vi "PiezoController main.vi"(10 "Top":refnum<queue>, 11 "Rotator":refnum<queue>) -> (3 "Ended":bool)   [LabVIEW 2022 SP3, in "SampleRotator.lvlib"]
doc: "This is a main VI of module for Sample rotator. It recives and executes commands, which comes from master controller. \nCommands and responses:\n\n/* */\nInitialize(path to driver DLL); -> Initialized(Contoller info<devN, devT, ID, Serial, Addr, connected?>);\n\n/* */\nUpdate(); -> Update(axis status<axis info, position, frequency, voltage>);\n\n/* */\nSetParameters(parameters<freq[Hz]; ampl[V]; offset[V]; tolerance[um]>); -> ParametersSet(parameters<freq; amp; offset; tolerance>);\n\n/* */\nSetPositon(positionToSet<relative?, double>) -> PositionSet(position to set<relative?, doubele);\n\n/* */\nEnd(), -> Disconnected();"
uses:
  SampleRotator.lvlib
  ctl/Rotator all.ctl
  ctl/Axis status.ctl
  Messenger service/Data types/Module name.ctl
  ctl/Motion Properties.ctl
  ctl/Positoin to set.ctl
  ctl/Rotator commands.ctl
panel:
  out "Piezo\nstatus":T1 {"Axes"."Index" items=["1", "2", "3"]; "Axes"."ActuatorType" items=["Linear", "Rotator", "Goniometer"]; "Features" format="%08b"; "FW-Version" format="%x"; "Controller info"."DeviceType" items=["ANC350res", "ANC350num", "ANC350fps", "No device / invalid"]; "Controller info"."ID" format="%x"}
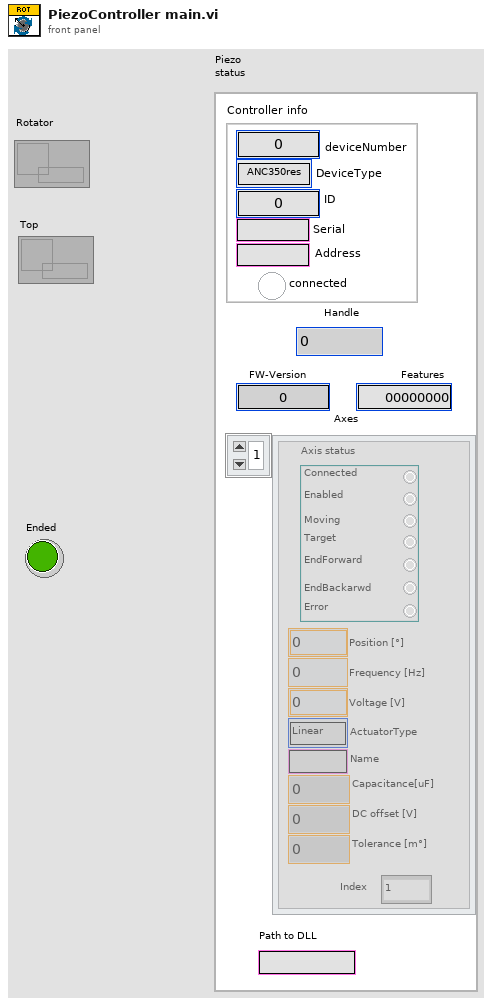
[diagram p1: front panel]
types:
  T1 = typedef "SampleRotator.lvlib/Rotator all.ctl" = cluster{"Controller info":cluster{"deviceNumber":i32, "DeviceType":i32, "ID":u32, "Serial":string, "Address":string, "connected":bool}, "Handle":u64, "FW-Version":i32, "Features":u32, "Axes":T2[], "Path to DLL":path}
  T2 = typedef "SampleRotator.lvlib/Axis status.ctl" = cluster{"Axis status":cluster{"Connected":bool, "Enabled":bool, "Moving":bool, "Target":bool, "EndForward":bool, "EndBackarwd":bool, "Error":bool}, "Position [°]":dbl, "Frequency [Hz]":dbl, "Voltage [V]":dbl, "Capacitance[uF]":dbl, "Name":string, "ActuatorType":u16, "DC offset [V]":dbl, "Tolerance [m°]":dbl, "Index":u8}
  T3 = typedef "SampleRotator.lvlib/Rotator commands.ctl" = enum16{"Ignore", "Initialize", "Initialize axes", "Update", "Set parameters", "Stop movement", "Set position", "Disconnect", "End"}
  T4 = typedef "Module name.ctl" = enum16{"Emty", "Magnet", "VTI", "Excitation", "Servo", "Acquisition", "Rotator", "Digitizer", "SMU2450", "Carousel", "Multimeter", "Tmp monitor", "Power monitor"}
  T5 = typedef "Motion Properties.ctl" = cluster{"Frequency [Hz]":dbl, "MaxErr [µm|m°]":dbl, "DC voltage [V]":dbl, "Amplitude [V]":dbl, "Position [mm|°]":dbl, "EoF":bool, "EoB":bool, "Error":bool, "Target [mm|°]":dbl}
  T6 = typedef "Positoin to set.ctl" = cluster{"Relative?":bool, "Position [°]":dbl, "Safe to move?":bool}
  T7 = cluster{"deviceNumber":i32, "DeviceType":i32, "ID":u32, "Serial":string, "Address":string, "connected":bool}
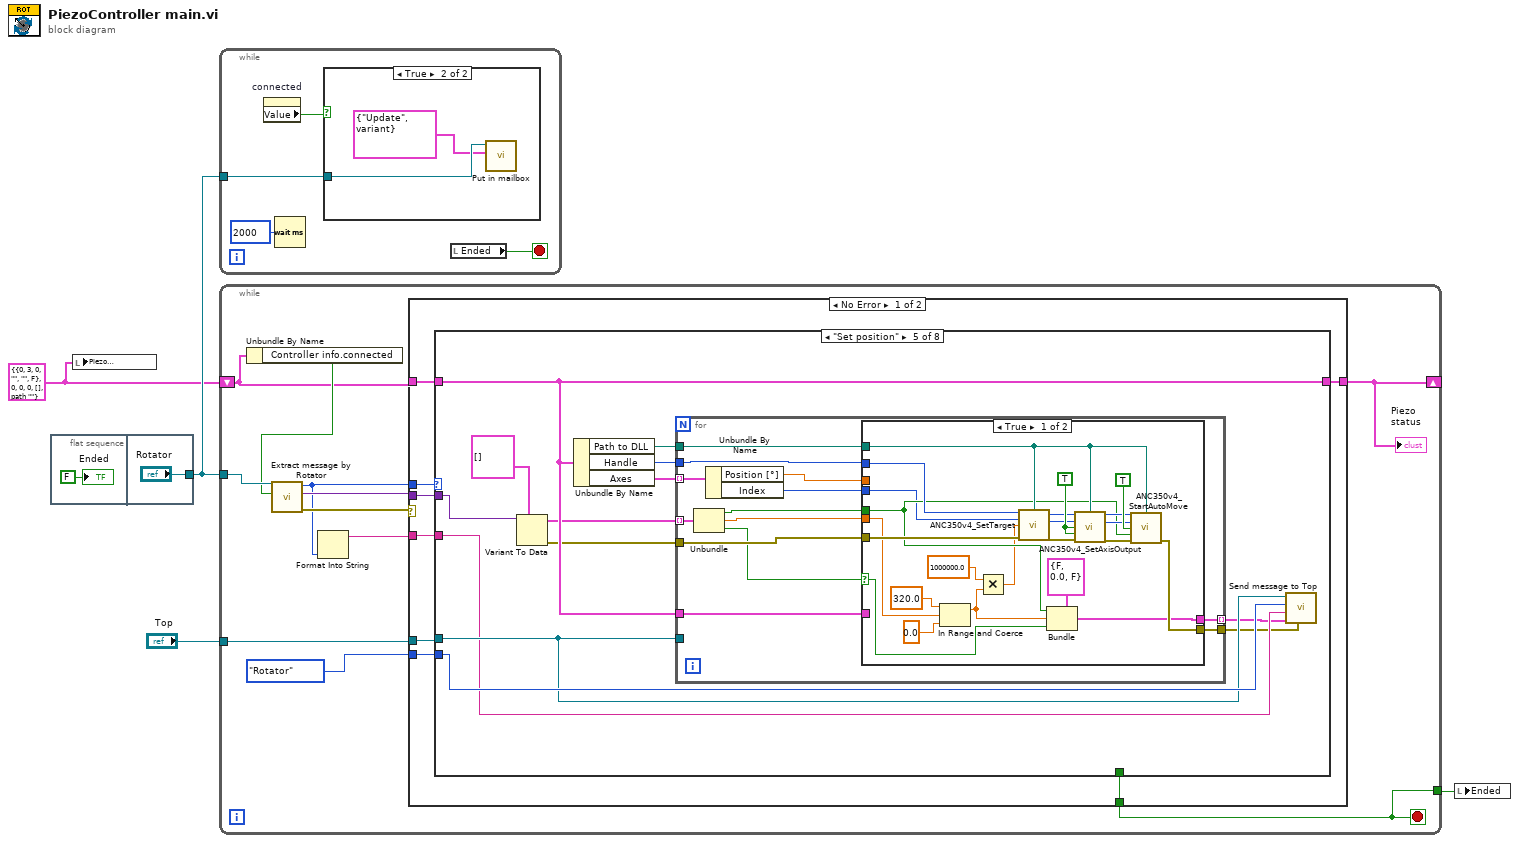
[diagram p0: block diagram]
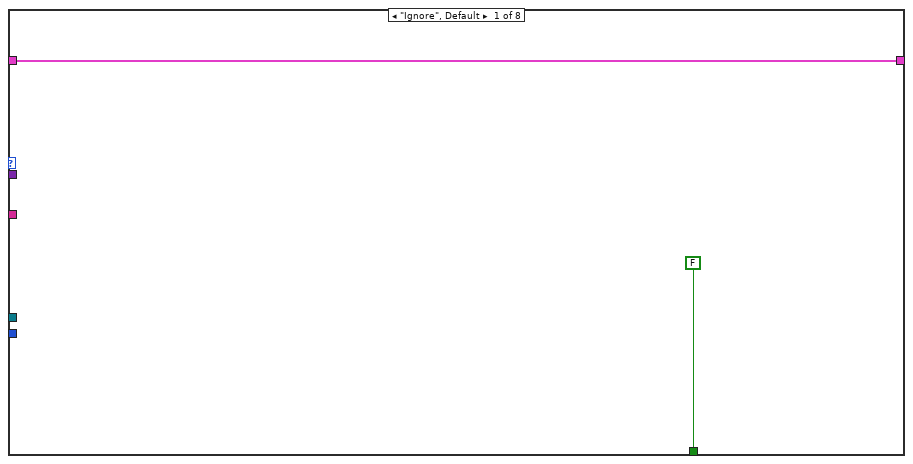
[diagram p3: hidden frame]
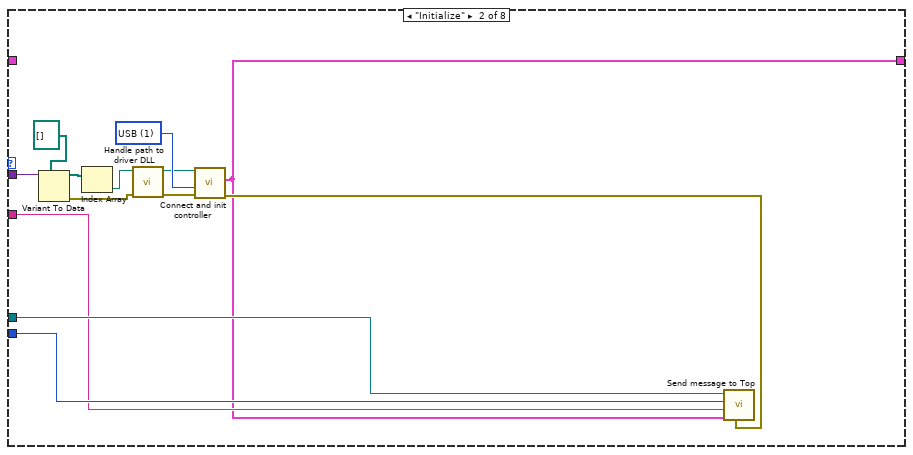
[diagram p4: hidden frame]
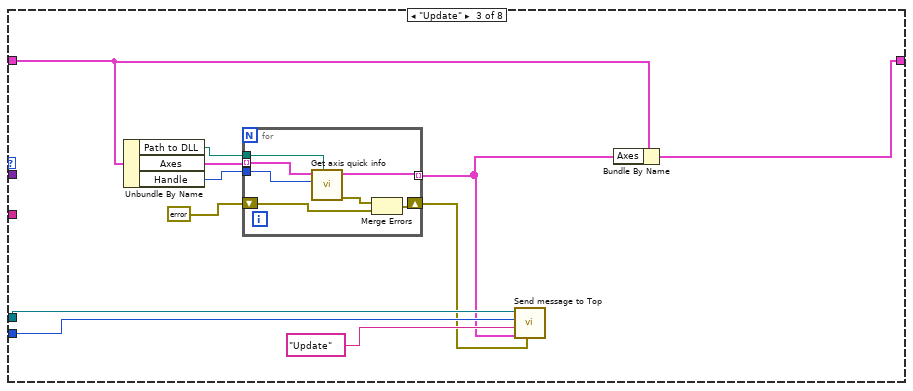
[diagram p5: hidden frame]
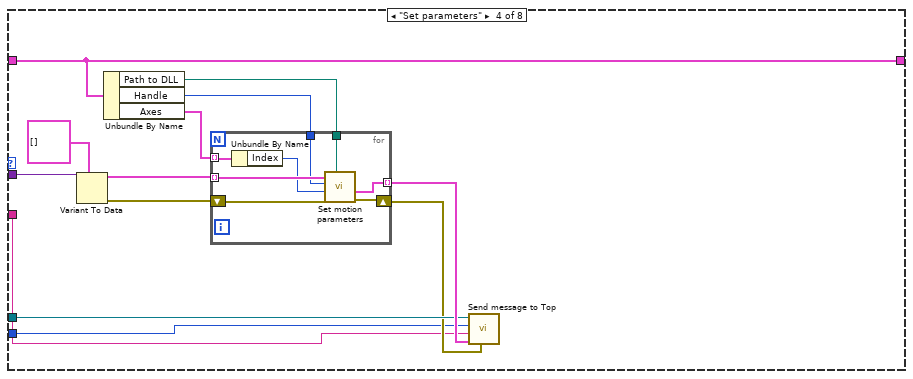
[diagram p6: hidden frame]
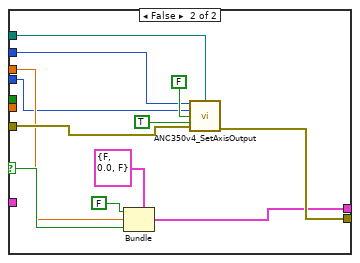
[diagram p7: hidden frame]
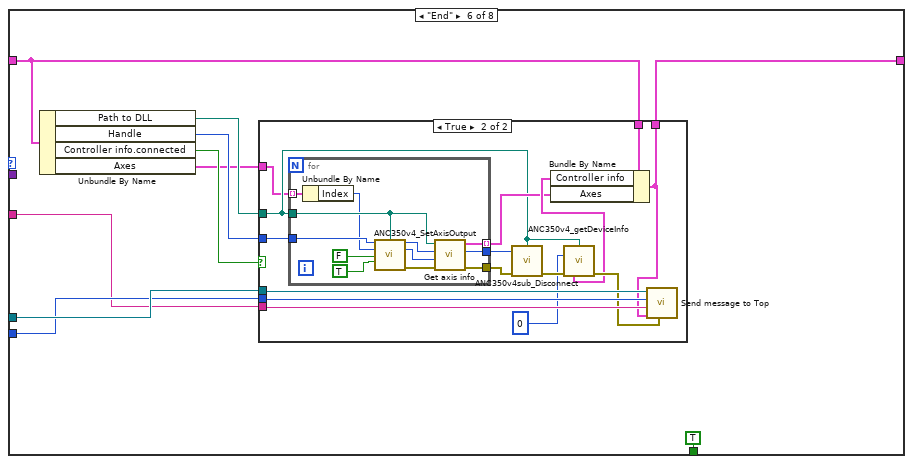
[diagram p8: hidden frame]
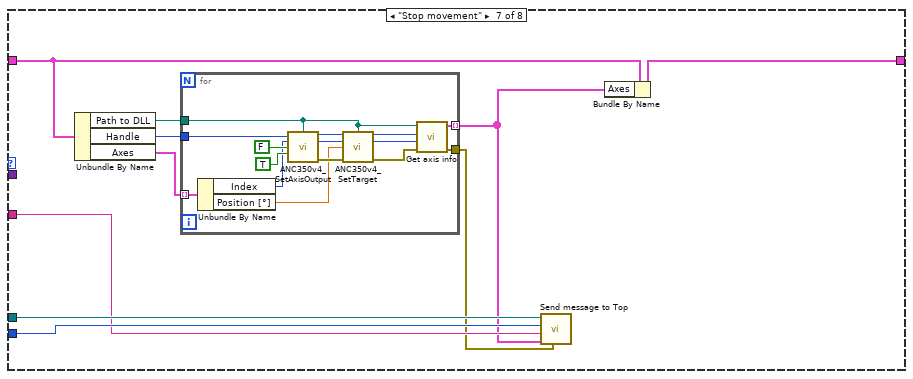
[diagram p10: hidden frame]
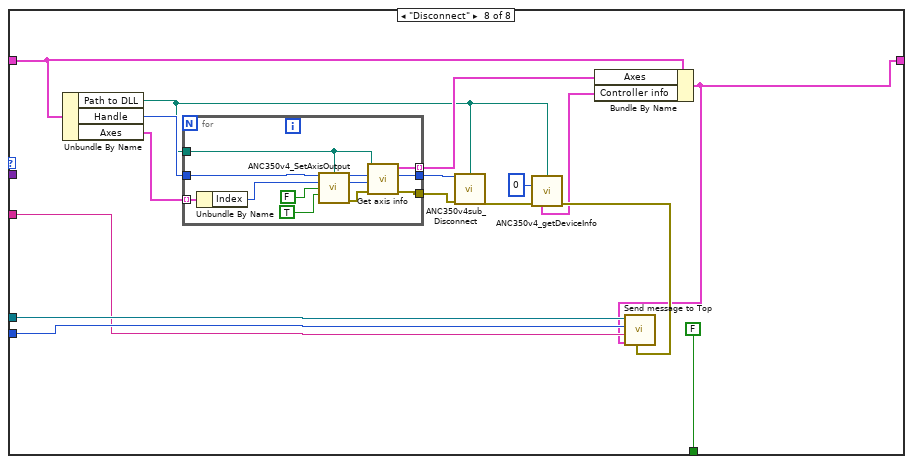
[diagram p11: hidden frame]
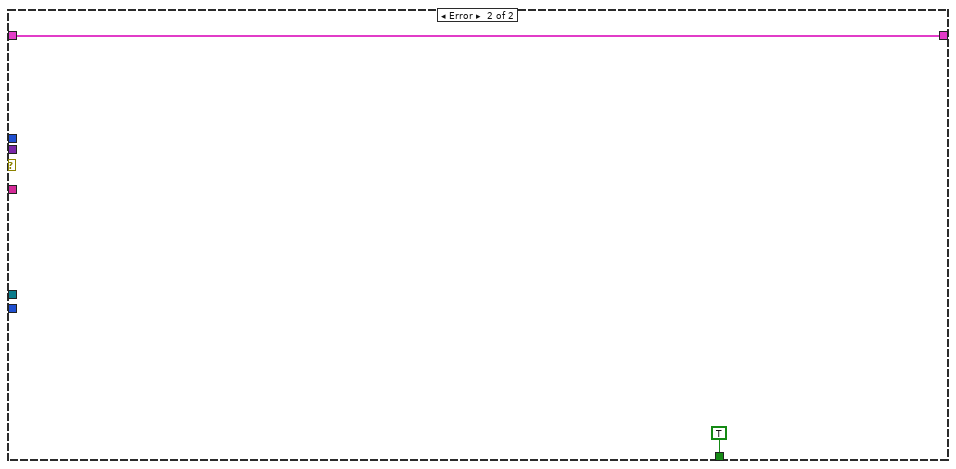
[diagram p12: hidden frame]
diagram:
  w1 = T1 {"Controller info"={"deviceNumber"=0, "DeviceType"=3, "ID"=0, "Serial"="", "Address"="", "connected"=FALSE}, "Handle"=0, "FW-Version"=0, "Features"=0, "Axes"=[], "Path to DLL"=path ""} ("Rotator")
  n1 = flat-sequence {
    tunnel: ["Rotator"] -> w2
    frame #0 {
      "Ended" <- FALSE
    }
    frame #1 {
    }
  }
  n2 = local write "Piezo\nstatus"(w1) -> ()
  n3 = while {
    tunnel: w2 -> [w7]
    stop <- w9 stop-if-true
    n4 = property on="connected" class="Bool (strict)"() -> ("Value"=w8:bool)  [unwired: 2 in, 2 out]
    n5 = Wait (ms)(milliseconds to wait=u32 2000) -> ()  [unwired: 1 out]
    n6 = case shown="True" w8 {
      tunnel: w7 -> [_ w12]
      frame False {
      }
      frame True {
        n7 = call "Put in mailbox.vi"("Message"=cluster{"Command":T3, "Data":variant} {"Command"=enum."Update", "Data"=variant} ("MSG to rotator"), "Queue in"=w12) -> ()  [unwired: 7 in, 3 out]
      }
    }
    n8 = local read "Ended"() -> (w9:bool)
  }
  n9 = while {
    tunnel: "Top" -> [w23]
    shift-right: [w20] -> _
    shift-left: w1 -> [w14]
    tunnel: [w16] -> w3
    tunnel: w2 -> [w17]
    stop <- w16 stop-if-true
    n10 = Unbundle By Name(w14) -> ("Controller info.connected"=w15:bool)
    n11 = call "Extract message by Rotator.vi"("Initialized?"=w15, "Queue in"=w17) -> ("error out"=w18:errorcluster, "Data"=w21:variant, "Command out"=w13:T3)  [unwired: 6 in, 1 out]
    n12 = Format Into String(w13) -> (resulting string=w19:string)  [unwired: 3 in, 1 out]
    n13 = case shown="No Error" w18 {
      tunnel: w23 -> [w31 _]
      tunnel: Module_name."Rotator" ("Module name") -> [w30 _]
      tunnel: w21 -> [w29 _]
      tunnel: [w28 w238] -> w20
      tunnel: w14 -> [w27 w238]
      tunnel: [w26 TRUE] -> w16
      tunnel: w13 -> [w25 _]
      tunnel: w19 -> [w24 _]
      frame No Error {
        n14 = case shown="\"Set position\"" w25 {
          tunnel: [FALSE _ _ _ _ TRUE _ FALSE] -> w26
          tunnel: w31 -> [_ w46 w57 w73 w92 w156 w194 w225]
          tunnel: w30 -> [_ w45 w56 w71 w93 w155 w193 w224]
          tunnel: w29 -> [_ w44 _ w75 w98 _ _ _]
          tunnel: [w32 w36 w51 w68 w96 w148 w188 w213] -> w28
          tunnel: w27 -> [w32 _ w52 w68 w96 w149 w191 w221]
          tunnel: w24 -> [_ w40 _ w70 w91 w153 w192 w222]
          frame "Ignore", Default {
          }
          frame "Initialize" {
            w39 = u32 1 items=["None", "USB", "TCP", "All"] ("Interface types")
            n15 = Variant To Data(type=path[] [], Variant=w44) -> (data=w42:path[], error out=w34:errorcluster)  [unwired: 1 in]
            n16 = Index Array(array=w42) -> (element=w38:path)  [unwired: 1 in]
            n17 = call "Handle path to driver DLL.vi"("error in (no error)"=w34, "Path to DLL"=w38) -> ("error out"=w41:errorcluster, "path out"=w35:path)  [unwired: 8 in]
            n18 = call "Connect and init controller.vi"("error in (no error)"=w41, "Interface types"=w39, "path to dll"=w35) -> ("error out"=w37:errorcluster, "Rotator"=w36:T1)  [unwired: 7 in]
            n19 = call "Send message to Top.vi"("Error in (no error)"=w37, "Data"=w36, "Response"=w40, "Module"=w45, "Mailbox address in"=w46) -> ()  [unwired: 5 in, 2 out]
          }
          frame "Update" {
            n20 = Unbundle By Name(w52) -> ("Path to DLL"=w53:path, "Axes"=w48:T2[], "Handle"=w49:u64)
            n21 = for {
              tunnel: w53 -> [w61]
              tunnel: w49 -> [w60]
              tunnel: [w63] -> w50 mode=indexing
              tunnel: w48 -> [w62] mode=indexing
              shift-right: [w59] -> w54
              shift-left: errorcluster {"status"=FALSE, "code"=0, "source"=""} ("error IO") -> [w58]
              n22 = call "Get axis quick info.vi"("path in"=w61, "deviceHandle"=w60, "Axis status in"=w62) -> ("error out"=w64:errorcluster, "Axis status"=w63:T2)  [unwired: 5 in, 2 out]
              n23 = Merge Errors(w64, w58) -> (w59:errorcluster)
            }
            n24 = call "Send message to Top.vi"("Error in (no error)"=w54, "Data"=w50, "Response"="Update", "Module"=w56, "Mailbox address in"=w57) -> ()  [unwired: 5 in, 2 out]
            n25 = Bundle By Name(cluster=w52, "Axes"=w50) -> (w51:T1)
          }
          frame "Set parameters" {
            n26 = Variant To Data(type=T5[] [] ("Motion parameters"), Variant=w75) -> (data=w77:T5[], error out=w76:errorcluster)  [unwired: 1 in]
            n27 = Unbundle By Name(w68) -> ("Path to DLL"=w66:path, "Handle"=w67:u64, "Axes"=w65:T2[])
            n28 = for {
              tunnel: w67 -> [w81]
              tunnel: w66 -> [w80]
              shift-right: [w82] -> w72
              shift-left: w76 -> [w84]
              tunnel: w77 -> [w85] mode=indexing
              tunnel: [w83] -> w74 mode=indexing
              tunnel: w65 -> [w79] mode=indexing
              n29 = Unbundle By Name(w79) -> ("Index"=w78:u8)
              n30 = call "Set motion parameters.vi"("path in"=w80, "error in (no error)"=w84, "axis in"=w78, "deviceHandle in"=w81, "Motion parameters"=w85) -> ("error out"=w82:errorcluster, "Motion parameters out"=w83:T5)  [unwired: 3 in, 2 out]
            }
            n31 = call "Send message to Top.vi"("Error in (no error)"=w72, "Data"=w74, "Response"=w70, "Module"=w71, "Mailbox address in"=w73) -> ()  [unwired: 5 in, 2 out]
          }
          frame "Set position" {
            n32 = Variant To Data(type=T6[] [], Variant=w98) -> (data=w95:T6[], error out=w94:errorcluster)  [unwired: 1 in]
            n33 = Unbundle By Name(w96) -> ("Path to DLL"=w88:path, "Handle"=w89:u64, "Axes"=w90:T2[])
            n34 = for {
              tunnel: w96 -> [w111]
              tunnel: w95 -> [w110] mode=indexing
              tunnel: w94 -> [w109]
              tunnel: w92 -> [_]
              tunnel: w90 -> [w105] mode=indexing
              tunnel: w89 -> [w104]
              tunnel: w88 -> [w103]
              tunnel: [w101] -> w87
              tunnel: [w100] -> w86 mode=indexing
              n35 = Unbundle(w110) -> ("Relative?"=w108:bool, "Position [°]"=w107:dbl, "Safe to move?"=w106:bool)
              n36 = Unbundle By Name(w105) -> ("Position [°]"=w102:dbl, "Index"=w99:u8)
              n37 = case shown="True" w106 {
                selector: w106 -> [w119 w143]
                tunnel: w111 -> [_ _]
                tunnel: w109 -> [w126 w144]
                tunnel: w108 -> [w114 _]
                tunnel: w107 -> [w121 _]
                tunnel: w102 -> [_ w139]
                tunnel: w104 -> [w118 w140]
                tunnel: w103 -> [w117 w142]
                tunnel: [w116 w137] -> w101
                tunnel: [w115 w136] -> w100
                tunnel: w99 -> [w113 w135]
                frame True {
                  w133 = TRUE ("autoDisable")
                  n38 = In Range and Coerce(upper limit=320.0 ("lower limit"), x=w121, lower limit=0.0 ("upper limit")) -> (coerced(x)=w122:dbl)  [unwired: 1 out]
                  n39 = Multiply(x=1000000.0, y=w122) -> (x*y=w112:dbl)
                  n40 = call <instrlib>:"ANC350v4_SetTarget.vi"("deviceHandle"=w118, "Path to *.DLL"=w117, "axis"=w113, "Target [µm | m°]"=w112, "error in"=w126) -> ("deviceHandle"=w128:u64, "axis"=w127:u8, "error ANC350v4_setTarget"=w132:errorcluster)  [unwired: 8 in]
                  n41 = Bundle(cluster=T6 {"Relative?"=FALSE, "Position [°]"=0.0, "Safe to move?"=FALSE}, "Relative?"=w114, "Position [°]"=w122, "Safe to move?"=w119) -> (w115:T6)
                  n42 = call <instrlib>:"ANC350v4_SetAxisOutput.vi"("deviceHandle"=w128, "Path to *.DLL"=w117, "axis"=w127, "enable"=w133, "autoDisable"=w133, "error in"=w132) -> ("deviceHandle"=w130:u64, "axis"=w129:u8, "error ANC350v4_setAxisOutput"=w131:errorcluster)  [unwired: 7 in]
                  n43 = call <instrlib>:"ANC350v4_StartAutoMove.vi"("deviceHandle"=w130, "Path to *.DLL"=w117, "axis"=w129, "Enable | Disable"=TRUE, "Relative | Absolute"=w114, "error in"=w131) -> ("error ANC350v4_StartAutoMove"=w116:errorcluster)  [unwired: 7 in, 2 out]
                }
                frame False {
                  n44 = Bundle(cluster=T6 {"Relative?"=FALSE, "Position [°]"=0.0, "Safe to move?"=FALSE}, "Relative?"=FALSE, "Position [°]"=w139, "Safe to move?"=w143) -> (w136:T6)
                  n45 = call <instrlib>:"ANC350v4_SetAxisOutput.vi"("deviceHandle"=w140, "Path to *.DLL"=w142, "axis"=w135, "enable"=FALSE ("autoDisable"), "autoDisable"=TRUE, "error in"=w144) -> ("error ANC350v4_setAxisOutput"=w137:errorcluster)  [unwired: 7 in, 2 out]
                }
              }
            }
            n46 = call "Send message to Top.vi"("Error in (no error)"=w87, "Data"=w86, "Response"=w91, "Module"=w93, "Mailbox address in"=w92) -> ()  [unwired: 5 in, 2 out]
          }
          frame "End" {
            n47 = Unbundle By Name(w149) -> ("Path to DLL"=w152:path, "Handle"=w151:u64, "Controller info.connected"=w150:bool, "Axes"=w147:T2[])
            n48 = case shown="True" w150 {
              tunnel: w156 -> [_ w172]
              tunnel: w155 -> [_ w171]
              tunnel: w153 -> [_ w170]
              tunnel: w152 -> [_ w160]
              tunnel: w151 -> [_ w169]
              tunnel: w149 -> [w157 w165]
              tunnel: [w157 w159] -> w148
              tunnel: w147 -> [_ w158]
              frame False {
              }
              frame True {
                n49 = for {
                  tunnel: [w182] -> w163
                  tunnel: [w181] -> w162 mode=indexing
                  tunnel: w160 -> [w177]
                  tunnel: w169 -> [w184]
                  tunnel: [w180] -> w161
                  tunnel: w158 -> [w174] mode=indexing
                  n50 = Unbundle By Name(w174) -> ("Index"=w173:u8)
                  n51 = call <instrlib>:"ANC350v4_SetAxisOutput.vi"("deviceHandle"=w184, "Path to *.DLL"=w177, "axis"=w173, "enable"=FALSE, "autoDisable"=TRUE) -> ("deviceHandle"=w178:u64, "axis"=w179:u8, "error ANC350v4_setAxisOutput"=w183:errorcluster)  [unwired: 8 in]
                  n52 = call "Get axis info.vi"("error in"=w183, "axis"=w179, "deviceHandle"=w178, "path in"=w177) -> ("error out"=w182:errorcluster, "deviceHandle out"=w180:u64, "Axis info"=w181:T2)  [unwired: 4 in, 1 out]
                }
                n53 = call <instrlib>:"ANC350v4sub_Disconnect.vi"("ANC350v4_Handle"=w161, "Path to *.DLL"=w160, "error in"=w163) -> ("error ANC350v4_Dis/Connect"=w168:errorcluster)  [unwired: 12 in]
                n54 = call <instrlib>:"ANC350v4_getDeviceInfo.vi"("Path to *.DLL"=w160, "deviceNumber"=u32 0, "error in"=w168) -> ("output cluster"=w164:T7, "Error_ANC350v4_getDeviceInfo"=w167:errorcluster)  [unwired: 5 in, 6 out]
                n55 = Bundle By Name(cluster=w165, "Controller info"=w164, "Axes"=w162) -> (w159:T1)
                n56 = call "Send message to Top.vi"("Error in (no error)"=w167, "Data"=w159, "Response"=w170, "Module"=w171, "Mailbox address in"=w172) -> ()  [unwired: 5 in, 2 out]
              }
            }
          }
          frame "Stop movement" {
            n57 = Unbundle By Name(w191) -> ("Path to DLL"=w185:path, "Handle"=w190:u64, "Axes"=w186:T2[])
            n58 = for {
              tunnel: w190 -> [w209]
              tunnel: [w208] -> w189
              tunnel: [w207] -> w187 mode=indexing
              tunnel: w186 -> [w204] mode=indexing
              tunnel: w185 -> [w201]
              n59 = Unbundle By Name(w204) -> ("Index"=w195:u8, "Position [°]"=w196:dbl)
              n60 = call <instrlib>:"ANC350v4_SetAxisOutput.vi"("deviceHandle"=w209, "Path to *.DLL"=w201, "axis"=w195, "enable"=FALSE, "autoDisable"=TRUE) -> ("deviceHandle"=w203:u64, "axis"=w202:u8, "error ANC350v4_setAxisOutput"=w197:errorcluster)  [unwired: 8 in]
              n61 = call <instrlib>:"ANC350v4_SetTarget.vi"("deviceHandle"=w203, "Path to *.DLL"=w201, "axis"=w202, "Target [µm | m°]"=w196, "error in"=w197) -> ("deviceHandle"=w200:u64, "axis"=w199:u8, "error ANC350v4_setTarget"=w198:errorcluster)  [unwired: 8 in]
              n62 = call "Get axis info.vi"("error in"=w198, "axis"=w199, "deviceHandle"=w200, "path in"=w201) -> ("error out"=w208:errorcluster, "Axis info"=w207:T2)  [unwired: 4 in, 2 out]
            }
            n63 = call "Send message to Top.vi"("Error in (no error)"=w189, "Data"=w187, "Response"=w192, "Module"=w193, "Mailbox address in"=w194) -> ()  [unwired: 5 in, 2 out]
            n64 = Bundle By Name(cluster=w191, "Axes"=w187) -> (w188:T1)
          }
          frame "Disconnect" {
            n65 = Unbundle By Name(w221) -> ("Path to DLL"=w211:path, "Handle"=w220:u64, "Axes"=w210:T2[])
            n66 = for {
              tunnel: [w231] -> w218 mode=indexing
              tunnel: [w230] -> w217
              tunnel: w211 -> [w229]
              tunnel: w220 -> [w237]
              tunnel: [w232] -> w219
              tunnel: w210 -> [w227] mode=indexing
              n67 = Unbundle By Name(w227) -> ("Index"=w226:u8)
              n68 = call <instrlib>:"ANC350v4_SetAxisOutput.vi"("deviceHandle"=w237, "Path to *.DLL"=w229, "axis"=w226, "enable"=FALSE, "autoDisable"=TRUE) -> ("deviceHandle"=w235:u64, "axis"=w234:u8, "error ANC350v4_setAxisOutput"=w233:errorcluster)  [unwired: 8 in]
              n69 = call "Get axis info.vi"("error in"=w233, "axis"=w234, "deviceHandle"=w235, "path in"=w229) -> ("error out"=w230:errorcluster, "deviceHandle out"=w232:u64, "Axis info"=w231:T2)  [unwired: 4 in, 1 out]
            }
            n70 = call <instrlib>:"ANC350v4sub_Disconnect.vi"("ANC350v4_Handle"=w219, "Path to *.DLL"=w211, "error in"=w217) -> ("error ANC350v4_Dis/Connect"=w216:errorcluster)  [unwired: 12 in]
            n71 = call <instrlib>:"ANC350v4_getDeviceInfo.vi"("Path to *.DLL"=w211, "deviceNumber"=u32 0, "error in"=w216) -> ("output cluster"=w212:T7, "Error_ANC350v4_getDeviceInfo"=w214:errorcluster)  [unwired: 5 in, 6 out]
            n72 = Bundle By Name(cluster=w221, "Axes"=w218, "Controller info"=w212) -> (w213:T1)
            n73 = call "Send message to Top.vi"("Error in (no error)"=w214, "Data"=w213, "Response"=w222, "Module"=w224, "Mailbox address in"=w225) -> ()  [unwired: 5 in, 2 out]
          }
        }
      }
      frame Error {
      }
    }
    "Piezo\nstatus" <- w20
  }
  n74 = local write "Ended"(w3) -> ()
